vi "MB Ethernet Transmit.vi"(7 "MBAP Header":T1, 8 "error in (no error)":errorcluster, 10 "Modbus Data Unit":T2={"function"=1, "Data"=[]} {"function" items=["Read Discrete Inputs"=2, "Read Coils"=1, "Write Single Coil"=5, "Write Multiple Coils"=15, "Read Input Register"=4, "Read Holding Registers"=3, "Write Single Register"=6, "Write Multiple Registers"=16, "Read/Write Multiple Registers"=23, "Mask Write Register"=22, "Read FIFO Queue"=24, "Read File Record"=20, "Write File Record"=21, "Read Exception Status"=7, "Diagnostic"=8, "Get Com Event Counter"=11, "Get Com Event Log"=12, "Report Slave ID"=17, "Read Device Identification"=43]; "Data" format="%.0x"}, 11 "TCP in":refnum<class "TCP.lvclass">) -> (0 "error out":errorcluster, 3 "TCP out":refnum<class "TCP.lvclass">)   [LabVIEW 2019, in "NI_modbus_upd.lvlib"]
uses:
  Ctl/MB Modbus Data Unit.ctl
  Modbus Data Unit (PDU)/Function.ctl
  TCP/TCP.lvclass
  TCP/TCP.lvclass/TCP.ctl
  NI_modbus_upd.lvlib
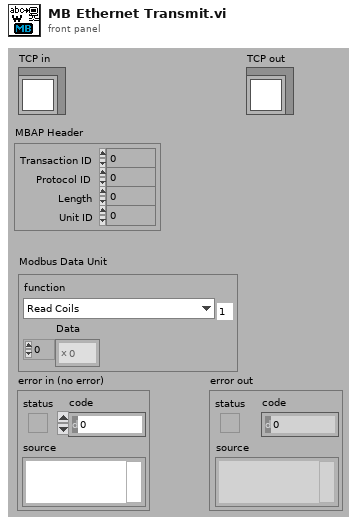
[diagram p1: front panel]
types:
  T1 = cluster{"Transaction ID":u16, "Protocol ID":u16, "Length":u16, "Unit ID":u8}
  T2 = typedef "NI_modbus_upd.lvlib/MB Modbus Data Unit.ctl" = cluster{"function":T3, "Data":u8[]}
  T3 = typedef "NI_modbus_upd.lvlib/Function.ctl" = u8
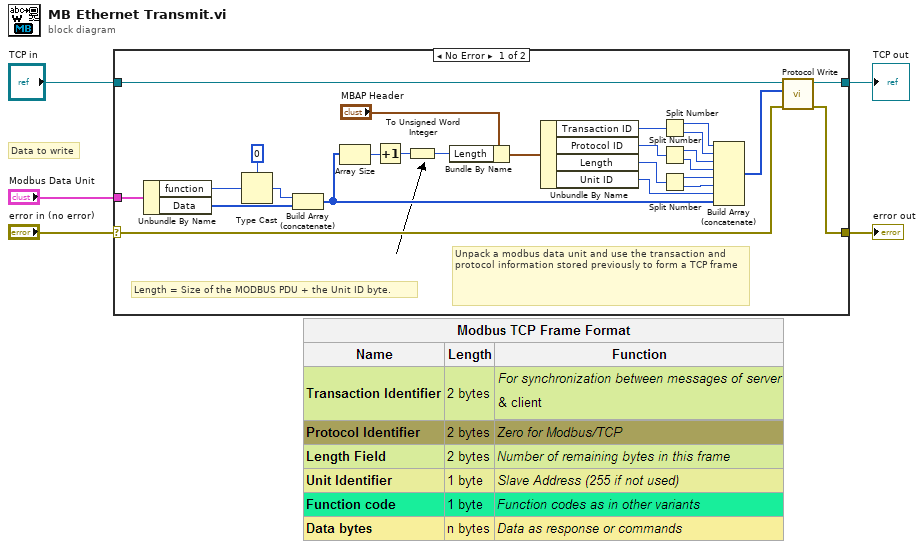
[diagram p0: block diagram]
diagram:
  # "Data to write"
  n1 = case shown="No Error" "error in (no error)" {
    selector: "error in (no error)" -> [w7 w33]
    tunnel: "Modbus Data Unit" -> [w31 _]
    tunnel: "TCP in" -> [w9 w32]
    tunnel: [w8 w32] -> w3
    tunnel: [w6 w33] -> w1
    frame No Error {
      # "Unpack a modbus data unit and use the transaction and protocol information stored previously to form a TCP frame"
      # "Length = Size of the MODBUS PDU + the Unit ID byte."
      n2 = Unbundle By Name(w31) -> ("function"=w28:T3, "Data"=w27:u8[])
      n3 = Type Cast(type=u8 0, x=w28) -> (*(type *) &x=w30:u8)
      n4 = Build Array (concatenate)(w30, w27) -> (w13:u8[])
      n5 = Array Size(array=w13) -> (size(s)=w17:i32)
      n6 = Increment(x=w17) -> (x+1=w16:i32)
      n7 = To Unsigned Word Integer(number=w16) -> (unsigned 16bit integer=w15:u16)
      n8 = Bundle By Name(cluster="MBAP Header", "Length"=w15) -> (w14:T1)
      n9 = Unbundle By Name(w14) -> ("Transaction ID"=w26:u16, "Protocol ID"=w25:u16, "Length"=w11:u16, "Unit ID"=w12:u8)
      n10 = Split Number(x=w26) -> (hi(x)=w24:u8, lo(x)=w23:u8)
      n11 = Split Number(x=w25) -> (hi(x)=w22:u8, lo(x)=w21:u8)
      n12 = Split Number(x=w11) -> (hi(x)=w20:u8, lo(x)=w19:u8)
      n13 = Build Array (concatenate)(w24, w23, w22, w21, w20, w19, w12, w13) -> (w10:u8[])
      n14 = call "Protocol Write.vi"("error in (no error)"=w7, "data"=w10, "protocol layer in"=w9) -> ("error out"=w6:errorcluster, "protocol layer out"=w8:refnum<class "TCP.lvclass">)  [unwired: 6 in, 1 out]
    }
    frame Error {
    }
  }
  "TCP out" <- w3
  "error out" <- w1
